vi "Configure GB.vi"(0 "VISA resource name":refnum<visa-resource-name>, 1 "Test Current (A)":string, 2 "Dwell Time (s)":string, 3 "Min GB Limit (ohm)":string, 4 "Max GB Limit (ohm)":string, 5 "error in (no error)":errorcluster, 7 "Command Terminator":bool=TRUE) -> (14 "VISA resource name out":refnum<visa-resource-name>, 15 "Command Output":string, 17 "Error Message":string, 18 "Error Code":i32, 19 "error out":errorcluster)   [LabVIEW 2010, in "VITREK V7X.lvlib"]
doc: "Configures the <b>GB</b> input.\n\n<b>Note:</b> please refer to the instrument manual for the <b>GB</b> input specification."
uses:
  VITREK V7X.lvlib
panel:
  # "Yes\n\nNo"
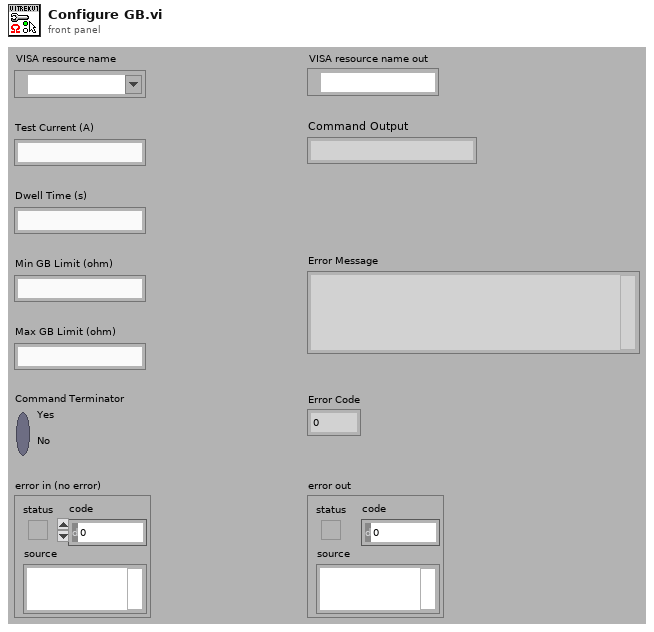
[diagram p1: front panel]
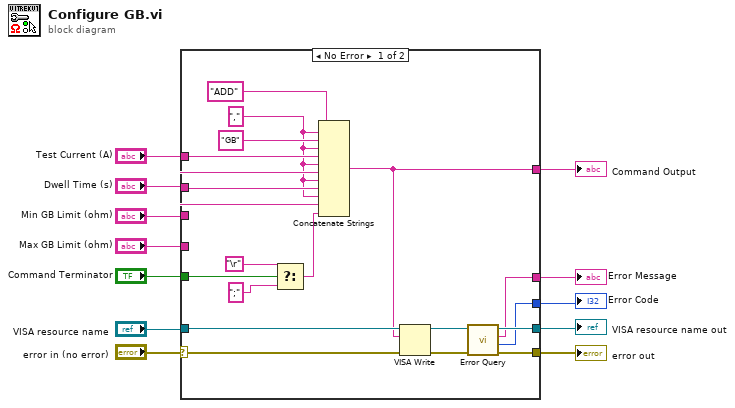
[diagram p0: block diagram]
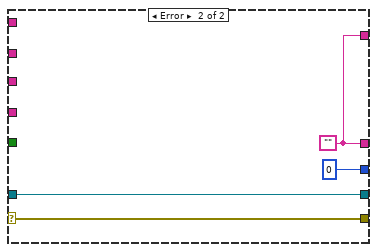
[diagram p2: hidden frame]
diagram:
  n1 = case shown="No Error" "error in (no error)" {
    selector: "error in (no error)" -> [w27 w35]
    tunnel: "VISA resource name" -> [w32 w36]
    tunnel: [w21 w34] -> w11
    tunnel: [w29 w36] -> w10
    tunnel: [w28 w35] -> w9
    tunnel: "Test Current (A)" -> [w26 _]
    tunnel: "Dwell Time (s)" -> [w25 _]
    tunnel: "Min GB Limit (ohm)" -> [w24 _]
    tunnel: "Max GB Limit (ohm)" -> [w23 _]
    tunnel: "Command Terminator" -> [w20 _]
    tunnel: [w14 0 ("Error Code")] -> w2
    tunnel: [w13 w34] -> w1
    frame No Error {
      w16 = ","
      n2 = Select(t="\r", s=w20, f=";") -> (s? t:f=w15:string)
      n3 = Concatenate Strings("ADD", w16, "GB", w16, w26, w16, w25, w16, w24, w16, w23, w15) -> (w21:string)
      n4 = VISA Write(VISA resource name=w32, write buffer=w21, error in (no error)=w27) -> (VISA resource name out=w31:refnum<visa-resource-name>, error out=w30:errorcluster)  [unwired: 1 out]
      n5 = call "Error Query.vi"("error in (no error)"=w30, "VISA resource name"=w31) -> ("error out"=w28:errorcluster, "Error Code"=w14:i32, "Error Message"=w13:string, "VISA resource name out"=w29:refnum<visa-resource-name>)  [unwired: 6 in]
    }
    frame Error {
      w34 = ""
    }
  }
  "VISA resource name out" <- w10
  "error out" <- w9
  "Command Output" <- w11
  "Error Code" <- w2
  "Error Message" <- w1
